vi "Self-Test.vi"(8 "error in (no error)":errorcluster, 11 "VISA resource name":refnum<visa-resource-name>) -> (0 "error out":errorcluster, 1 "Self-Test Result Message":string, 2 "Self-Test Result Code":i32, 3 "VISA resource name out":refnum<visa-resource-name>)   [LabVIEW 2018, in "JULABO DeviceDriver.lvlib"]
doc: "Runs the instrument's self-test routine and returns the test results."
uses:
  JULABO DeviceDriver.lvlib
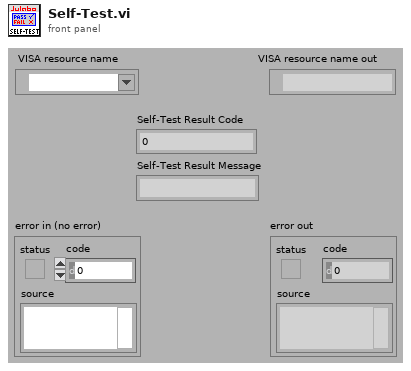
[diagram p1: front panel]
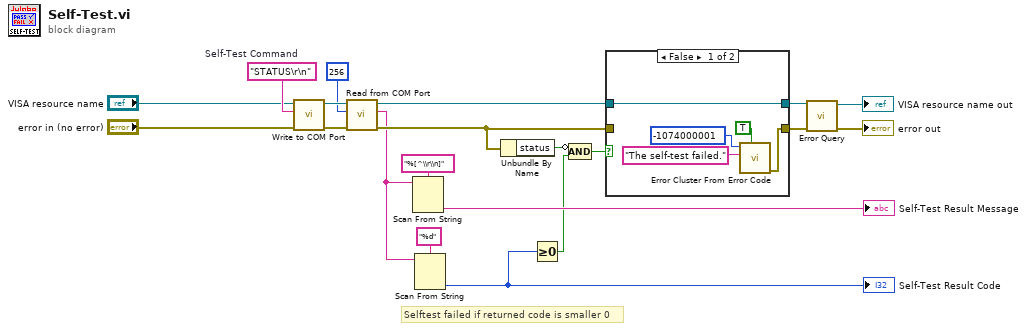
[diagram p0: block diagram]
diagram:
  w12 = "STATUS\r\n"  # Self-Test Command
  # "Selftest failed if returned code is smaller 0"
  n1 = call "Write to COM Port.vi"("error in"="error in (no error)", "Command (input)"=w12, "VISA resource name in"="VISA resource name") -> ("error out"=w17:errorcluster, "VISA resource name out"=w18:refnum<visa-resource-name>)  [unwired: 7 in]
  n2 = call "Read from COM Port.vi"("error in"=w17, "Byte to Read (-1:All)"=u32 256 ("byte count (20)"), "VISA resource name in"=w18) -> ("error out"=w4:errorcluster, "String (output)"=w1:string, "VISA resource name out"=w3:refnum<visa-resource-name>)  [unwired: 5 in, 1 out]
  n3 = Scan From String(format string="%[^\\r\\n]" ("Format String"), input string=w1) -> (output 1=→"Self-Test Result Message":string)  [unwired: 3 in, 3 out]
  n4 = Scan From String(format string="%d", input string=w1) -> (output 1=w2:i32)  [unwired: 3 in, 3 out]
  "Self-Test Result Code" <- w2
  n5 = Unbundle By Name(w4) -> ("status"=w8:bool)
  n6 = Greater Or Equal To 0?(x=w2) -> (x >= 0?=w9:bool)
  n7 = Compound Arithmetic op=AND(invert w8, w9) -> (w7:bool)
  n8 = case shown="False" w7 {
    tunnel: w3 -> [w25 w27]
    tunnel: w4 -> [_ w26]
    tunnel: [w21 w26] -> w11
    tunnel: [w25 w27] -> w10
    frame False {
      n9 = call <vilib>:"Error Cluster From Error Code.vi"("show call chain? (False)"=TRUE, "error message (\"\")"="The self-test failed." ("Source (VI Name)"), "error code (0)"=-1074000001 ("Code")) -> ("error out"=w21:errorcluster)  [unwired: 6 in]
    }
    frame True {
    }
  }
  n10 = call "Error Query.vi"("error in (no error)"=w11, "VISA resource name"=w10) -> ("error out"=→"error out":errorcluster, "VISA resource name out"=→"VISA resource name out":refnum<visa-resource-name>)  [unwired: 6 in, 2 out]
